vi "0xE9_Cmd_get_description_one_parameter_type_telem_(SubVI).vi"(10 "NumberTelemParam":i32 format="%0d", 11 "String in":string) -> (3 "String out":string)   [LabVIEW 2017, in "LV_Unicorn.lvlib"]
uses:
  LV_Unicorn.lvlib
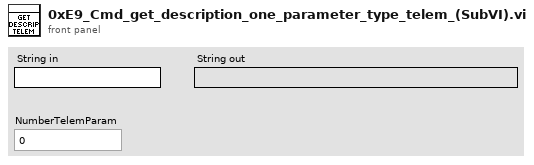
[diagram p1: front panel]
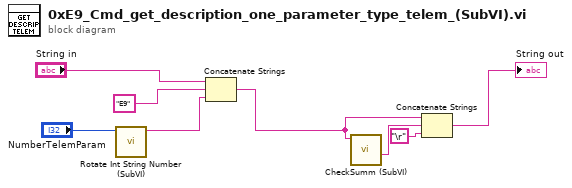
[diagram p0: block diagram]
diagram:
  n1 = call "Rotate Int String Number (SubVI).vi"("Int Number In"="NumberTelemParam") -> ("Orig String"=w2:string)  [unwired: 8 in, 2 out]
  n2 = Concatenate Strings("String in", "E9" ("string"), w2) -> (w3:string)
  n3 = call "CheckSumm (SubVI).vi"("Input String"=w3) -> ("CheckSumm"=w4:string)  [unwired: 7 in, 3 out]
  n4 = Concatenate Strings(w3, w4, "\r") -> (→"String out":string)
